vi "Setup PID.vi"(6 "Control Input":string, 7 "PID Params":T1={"P"=1.14, "I"=0.012, "D"=21.68, "Set"=0.0} {"D" min=0.0; "I" min=0.0; "P" min=0.0}, 8 "error in (no error)":errorcluster, 11 "VISA Refnum in":refnum<visa-resource-name>) -> (0 "error out":errorcluster, 3 "VISA Refnum out":refnum<visa-resource-name>)   [LabVIEW 2024]
uses:
  controls/PID Params.ctl
  Program Files/National Instruments/LabVIEW 2024/instr.lib/Stanford PTC10/SRS PTC10.lvlib
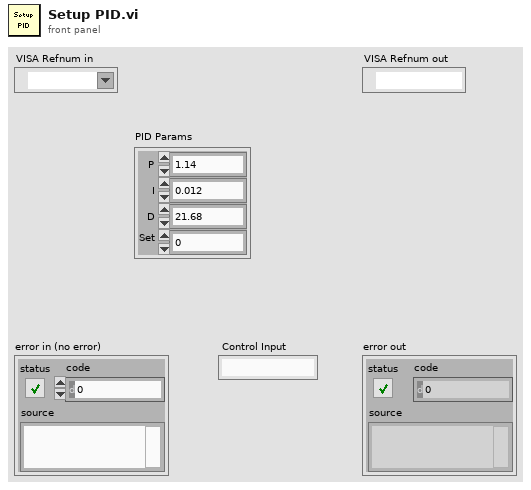
[diagram p1: front panel]
types:
  T1 = typedef "PID Params.ctl" = cluster{"P":dbl, "I":dbl, "D":dbl, "Set":dbl}
  T2 = enum8{"\"Input\"", "\"Set out\"", "\"Meas out\""}
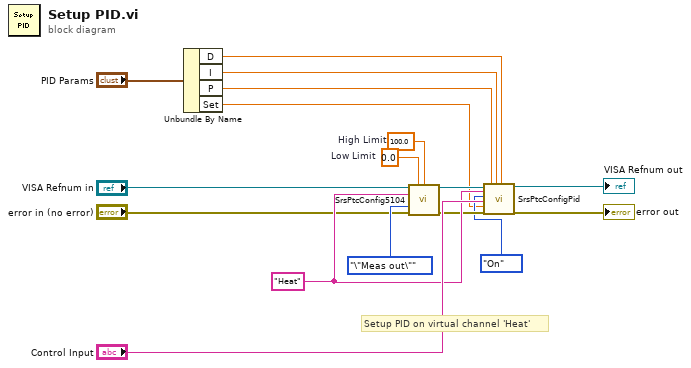
[diagram p0: block diagram]
diagram:
  w12 = 100.0  # High Limit
  w11 = 0.0  # Low Limit
  w13 = "Heat" ("Channel name")
  # "Setup PID on virtual channel 'Heat'"
  n1 = Unbundle By Name("PID Params") -> ("D"=w4:dbl, "I"=w3:dbl, "P"=w2:dbl, "Set"=w1:dbl)
  n2 = call "SrsPtcConfig5104.vi"("SRS PTC10 VISA in"="VISA Refnum in", "Low Limit"=w11, "High Limit"=w12, "Channel name"=w13, "I/O Type"=T2."\"Meas out\"", "error in"="error in (no error)") -> ("SRS PTC10 VISA out"=w10:refnum<visa-resource-name>, "error out"=w8:errorcluster)  [unwired: 7 in, 1 out]
  n3 = call "SrsPtcConfigPid.vi"("SRS PTC10 VISA in"=w10, "Channel name"=w13, "PID Mode"=enum16{"Off", "On"}."On", "Input channel name"="Control Input", "Setpoint"=w1, "error in"=w8, "P (proportional parameter)"=w2, "I (integral parameter)"=w3, "D (derivative parameter)"=w4) -> ("SRS PTC10 VISA out"=→"VISA Refnum out":refnum<visa-resource-name>, "error out"=→"error out":errorcluster)  [unwired: 8 in, 1 out]
